vi "GoAxis_complex2.vi"() -> ()   [LabVIEW 2020]
uses:
  <vilib>/Utility/error.llb/DialogType.ctl
panel:
  out "Index":i32=1 min=1 max=10
  in  "stop":bool
  out "axis moving":bool
  in  "set mode":bool
  in  "start":bool
  in  "exit":bool
  in  "Target mode":u32(ring) items=["relative", "absolute", "NDT", "PT30", "free", ""]
  in  "Target":i32
  out "Axis position":i32
  in  "Axis number":i32=1 min=1 max=3
  in  "Control unit ID":i32=1 min=1 max=10
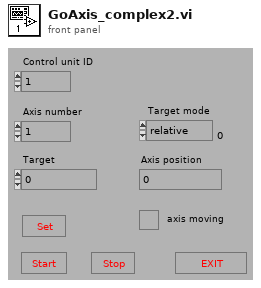
[diagram p1: front panel]
types:
  T1 = typedef "DialogType.ctl" = u16
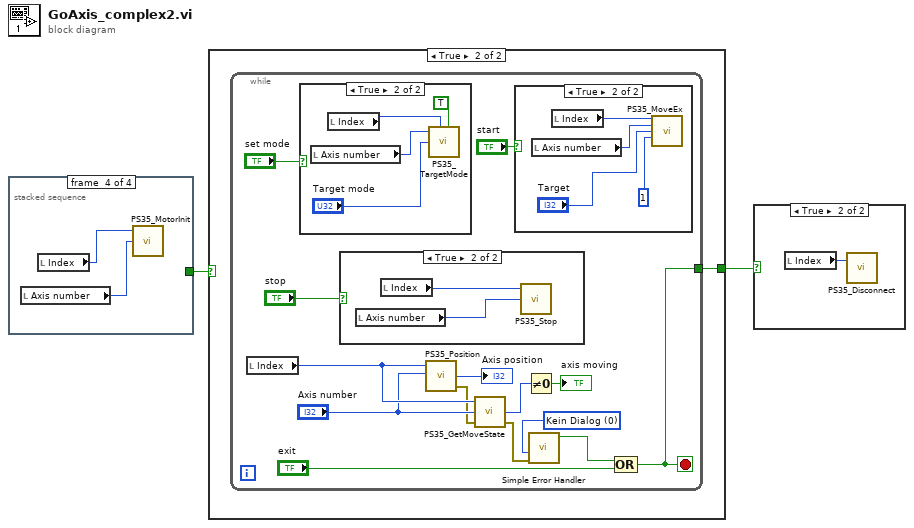
[diagram p0: block diagram]
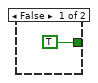
[diagram p3: hidden frame]
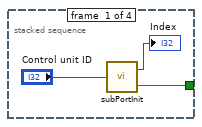
[diagram p7: hidden frame]
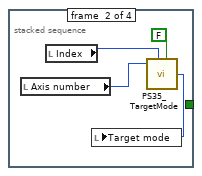
[diagram p8: hidden frame]
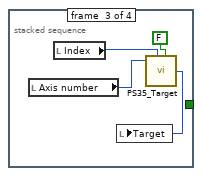
[diagram p9: hidden frame]
diagram:
  n1 = stacked-sequence {
    tunnel: [w4 _ _ _] -> w2
    frame #0 {
      n2 = call "subPortInit.vi"("Control unit ID"="Control unit ID") -> ("Index"=→"Index":i32, "InitOK"=w4:bool)
    }
    frame #1 {
      n3 = local read "Axis number"() -> (w7:i32)
      n4 = local read "Index"() -> (w8:i32)
      n5 = call "PS35_TargetMode.vi"("Axis number"=w7, "Control unit ID"=w8, "function"=FALSE) -> ("Value-Out"=w6:i32)  [unwired: 5 in, 1 out]
      n6 = local write "Target mode"(w6) -> ()
    }
    frame #2 {
      n7 = local read "Axis number"() -> (w13:i32)
      n8 = local read "Index"() -> (w12:i32)
      n9 = call "PS35_Target.vi"("Axis number"=w13, "Control unit ID"=w12, "function"=FALSE) -> ("Value-Out"=w10:i32)  [unwired: 5 in, 1 out]
      n10 = local write "Target"(w10) -> ()
    }
    frame #3 {
      n11 = local read "Axis number"() -> (w14:i32)
      n12 = local read "Index"() -> (w15:i32)
      n13 = call "PS35_MotorInit.vi"("Axis number"=w14, "Control unit ID"=w15) -> ()  [unwired: 2 in, 1 out]
    }
  }
  n14 = case shown="True" w2 {
    tunnel: [TRUE ("stop") w17] -> w1
    frame False {
    }
    frame True {
      n15 = while {
        tunnel: [w22] -> w17
        stop <- w22 stop-if-true
        w20 = T1 0 items=["Kein Dialog", "OK-Nachricht", "Dialog zum Fortsetzen oder Anhalten", "OK Nachricht + Warnungen", "Weiter/Stop + Warnung"] ("type of dialog (OK msg:1)")
        n16 = local read "Index"() -> (w27:i32)
        n17 = case shown="True" "set mode" {
          frame False {
          }
          frame True {
            n18 = local read "Axis number"() -> (w36:i32)
            n19 = local read "Index"() -> (w35:i32)
            n20 = call "PS35_TargetMode.vi"("Axis number"=w36, "Control unit ID"=w35, "Value-In"="Target mode", "function"=TRUE) -> ()  [unwired: 4 in, 2 out]
          }
        }
        n21 = case shown="True" "stop" {
          frame False {
          }
          frame True {
            n22 = local read "Axis number"() -> (w32:i32)
            n23 = local read "Index"() -> (w33:i32)
            n24 = call "PS35_Stop.vi"("Axis number"=w32, "Control unit ID"=w33) -> ()  [unwired: 2 in, 1 out]
          }
        }
        n25 = call "PS35_Position.vi"("Axis number"="Axis number", "Control unit ID"=w27) -> ("Value-Out"=→"Axis position":i32, "error out"=w23:errorcluster)  [unwired: 6 in]
        n26 = call "PS35_GetMoveState.vi"("error in (no error)"=w23, "Axis number"="Axis number", "Control unit ID"=w27) -> ("error out"=w19:errorcluster, "Move state"=w28:i32)  [unwired: 1 in]
        n27 = case shown="True" "start" {
          frame False {
          }
          frame True {
            n28 = local read "Axis number"() -> (w40:i32)
            n29 = local read "Index"() -> (w41:i32)
            n30 = call "PS35_MoveEx.vi"("Control unit ID"=w41, "Axis number"=w40, "dValue"="Target", "nEx"=1 ("bEx")) -> ()  [unwired: 11 in, 1 out]
          }
        }
        n31 = Not Equal To 0?(x=w28) -> (x != 0?=→"axis moving":bool)
        n32 = call <vilib>:"Simple Error Handler.vi"("type of dialog (OK msg:1)"=w20, "error in (no error)"=w19) -> ("error?"=w18:bool)  [unwired: 3 in, 4 out]
        n33 = Compound Arithmetic op=OR(w18, "exit") -> (w22:bool)
      }
    }
  }
  n34 = case shown="True" w1 {
    frame False {
    }
    frame True {
      n35 = local read "Index"() -> (w42:i32)
      n36 = call "PS35_Disconnect.vi"("Control unit ID"=w42) -> ()  [unwired: 2 in, 1 out]
    }
  }
